vi "H5Pget_userblock.vi"(6 "error in (no error)":errorcluster, 9 "HDF5 Property List Ref":T1) -> (0 "error out":errorcluster, 2 "size":u64, 3 "HDF5 Property List Ref out":T1)   [LabVIEW 2017]
doc: "Retrieves the size of a user block."
uses:
  <vilib>/UPVI/lvhdf5/library.llb/HDF5 Ref.ctl
  <vilib>/UPVI/lvhdf5/hdf5.dll
panel:
  # "LVHDF5 Toolkit\nCopyright (c) 2005-2013 by Jason D. Sommerville\nCopyright (c) 2014 by UPVI, LLC.\n\nThis use and distribution of this file is governed by the terms found in \nLICENSE.txt distributed with this toolkit and installed at\n <user.lib>\\_lvhdf5\\LICENSE.txt"
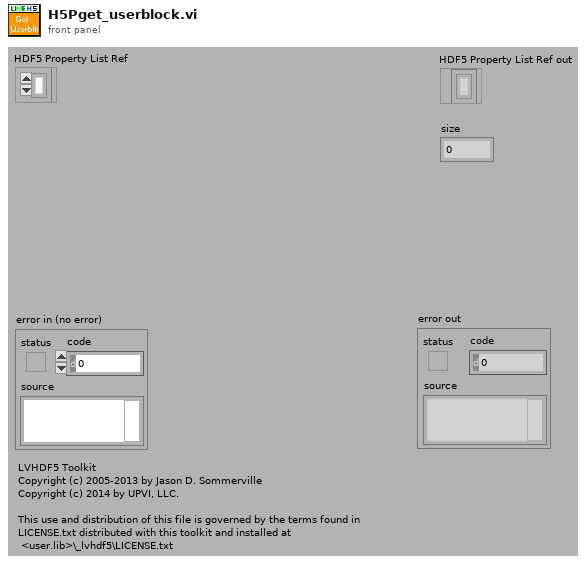
[diagram p1: front panel]
types:
  T1 = typedef "HDF5 Ref.ctl" = refnum<k1>
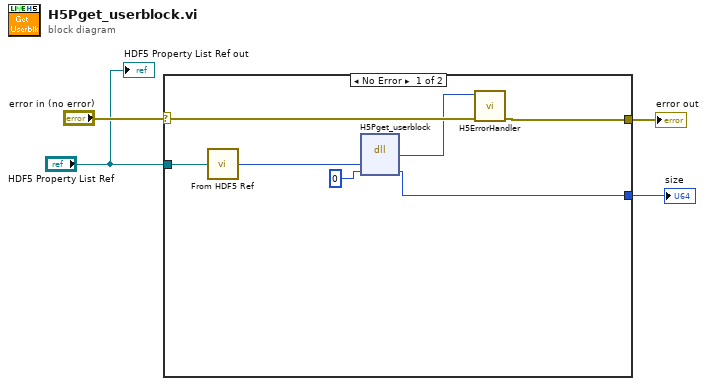
[diagram p0: block diagram]
diagram:
  n1 = case shown="No Error" "error in (no error)" {
    selector: "error in (no error)" -> [w11 w12]
    tunnel: [w6 w12] -> w3
    tunnel: "HDF5 Property List Ref" -> [w10 _]
    tunnel: [w5 _] -> w1
    frame No Error {
      n2 = call <vilib>:"From HDF5 Ref.vi"("HDF5 Ref"=w10) -> ("I32"=w9:i32)
      n3 = dll-call lib="C:/Program Files/National Instruments/LabVIEW 2017/vi.lib/UPVI/lvhdf5/hdf5.dll" fn="H5Pget_userblock"("plist_id"=w9, "size"=u64 0) -> ("return type"=w8:i32, "size"=w5:u64)  [unwired: 4 in, 2 out]
      n4 = call <vilib>:"H5ErrorHandler.vi"("error in (no error)"=w11, "herr_t"=w8) -> ("error out"=w6:errorcluster)  [unwired: 3 in, 4 out]
    }
    frame Error {
    }
  }
  "error out" <- w3
  "size" <- w1
  "HDF5 Property List Ref out" <- "HDF5 Property List Ref"
